vi "Get w4lvgrpc_ToClient.vi"(8 "error in (no error)":errorcluster, 11 "gRPCid":T1) -> (0 "error out":errorcluster, 2 "package_templatemessage":T2, 3 "gRPCid out":T1)   [LabVIEW 2019, in "Generated_server.lvlib"]
uses:
  Generated_server.lvlib
  2ed25e12-861d-4677-8ead-ace2906b2041.vi
  w4lvgrpc_ToClient_payload/w4lvgrpc_ToClient_payload.lvclass
  w4lvgrpc_ToClient.ctl
  w4lvgrpc_Msg_ToClient_1_Flat.ctl
  w4lvgrpc_Msg_ToClient_2_Flat.ctl
  w4lvgrpc_Msg_ToClient_3_Flat.ctl
  w4lvgrpc_Msg_ToClient_4_Flat.ctl
  w4lvgrpc_Msg_ToClient_5_Flat.ctl
  w4lvgrpc_Msg_ToClient_6_Flat.ctl
  w4lvgrpc_Msg_ToClient_7_Flat.ctl
  w4lvgrpc_Msg_ToClient_8_Flat.ctl
  w4lvgrpc_Msg_ToClient_9_Flat.ctl
  w4lvgrpc_ToClient_Flat.ctl
  <vilib>/gRPC/LabVIEW gRPC Library/Shared/grpcId.ctl
  <vilib>/gRPC/LabVIEW gRPC Library/grpc-lvsupport-release.lvlib
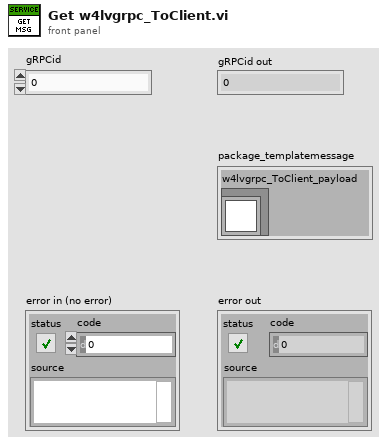
[diagram p1: front panel]
types:
  T1 = typedef "grpc-lvsupport-release.lvlib/grpcId.ctl" = u64
  T2 = typedef "Generated_server.lvlib/w4lvgrpc_ToClient.ctl" = cluster{"w4lvgrpc_ToClient_payload":refnum<class "w4lvgrpc_ToClient_payload.lvclass">}
  T3 = typedef "Generated_server.lvlib/w4lvgrpc_ToClient_Flat.ctl" = cluster{"w4lvgrpc_ToClient_payload_selected_index":i32, "msg_1":T4, "msg_2":T5, "msg_3":T6, "msg_4":T7, "msg_5":T8, "msg_6":T9, "msg_7":T10, "msg_8":T11, "msg_9":T12}
  T4 = typedef "Generated_server.lvlib/w4lvgrpc_Msg_ToClient_1_Flat.ctl" = cluster{"placeholder":string}
  T5 = typedef "Generated_server.lvlib/w4lvgrpc_Msg_ToClient_2_Flat.ctl" = cluster{"placeholder":string}
  T6 = typedef "Generated_server.lvlib/w4lvgrpc_Msg_ToClient_3_Flat.ctl" = cluster{"placeholder":string}
  T7 = typedef "Generated_server.lvlib/w4lvgrpc_Msg_ToClient_4_Flat.ctl" = cluster{"placeholder":string}
  T8 = typedef "Generated_server.lvlib/w4lvgrpc_Msg_ToClient_5_Flat.ctl" = cluster{"placeholder":string}
  T9 = typedef "Generated_server.lvlib/w4lvgrpc_Msg_ToClient_6_Flat.ctl" = cluster{"placeholder":string}
  T10 = typedef "Generated_server.lvlib/w4lvgrpc_Msg_ToClient_7_Flat.ctl" = cluster{"placeholder":string}
  T11 = typedef "Generated_server.lvlib/w4lvgrpc_Msg_ToClient_8_Flat.ctl" = cluster{"placeholder":string}
  T12 = typedef "Generated_server.lvlib/w4lvgrpc_Msg_ToClient_9_Flat.ctl" = cluster{"placeholder":string}
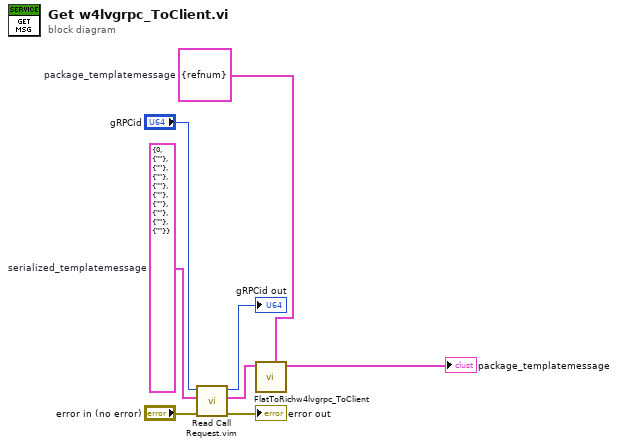
[diagram p0: block diagram]
diagram:
  w6 = T3 {"w4lvgrpc_ToClient_payload_selected_index"=0, "msg_1"={"placeholder"=""}, "msg_2"={"placeholder"=""}, "msg_3"={"placeholder"=""}, "msg_4"={"placeholder"=""}, "msg_5"={"placeholder"=""}, "msg_6"={"placeholder"=""}, "msg_7"={"placeholder"=""}, "msg_8"={"placeholder"=""}, "msg_9"={"placeholder"=""}}  # serialized_templatemessage
  w5 = T2 {"w4lvgrpc_ToClient_payload"=refnum}  # package_templatemessage
  n1 = call "Read Call Request.vim"("error in"="error in (no error)", "Request Type"=w6, "gRPCid in"="gRPCid") -> ("error out"=→"error out":errorcluster, "Request Data"=w4:T3, "gRPCid out"=→"gRPCid out":T1)  [unwired: 6 in]
  n2 = call "FlatToRichw4lvgrpc_ToClient.vi"("OutputClusterType"=w5, "InputCluster"=w4) -> ("OutputCluster"=→"package_templatemessage":T2)  [unwired: 9 in]
